vi "Split_Head_Tail.vi"(5 "Number of Cores":i32, 7 "Size":cluster{"X":i32, "Y":i32}, 9 "Major Angle":dbl, 10 "Centroid":cluster{"X":dbl, "Y":dbl}, 11 "Image Pixels (single)":sgl[][](array[numeric])) -> (1 "P2":sgl[][](array[numeric]), 2 "P1":sgl[][](array[numeric]), 3 "Split Line Points":cluster{"X":i32, "Y":i32}[](array[cluster]))   [LabVIEW 2014]
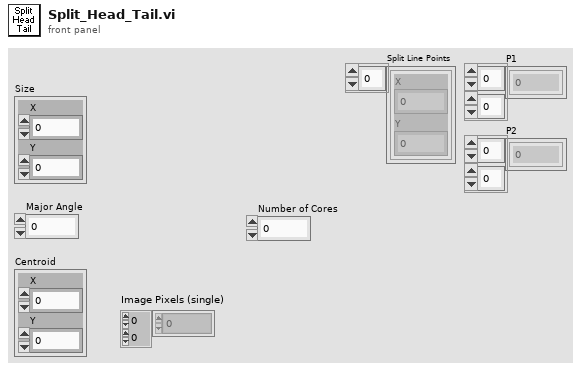
[diagram p1: front panel]
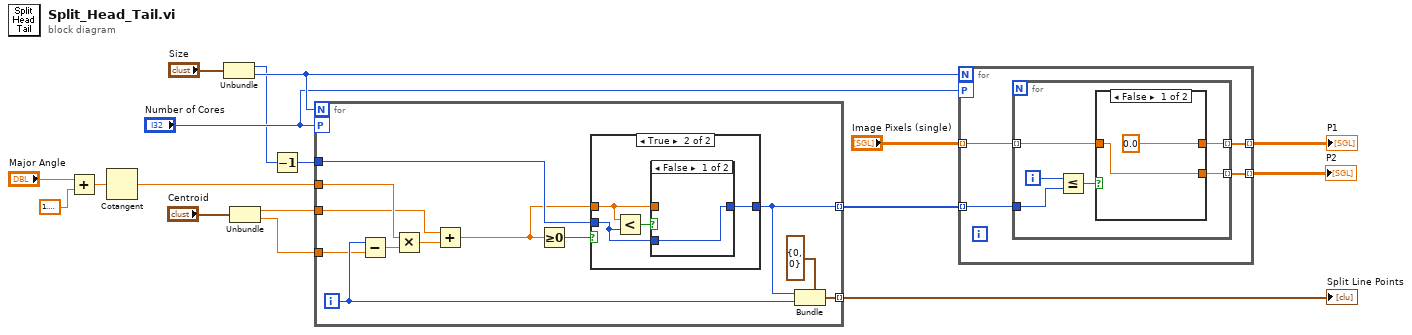
[diagram p0: block diagram]
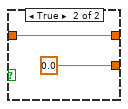
[diagram p2: hidden frame]
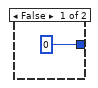
[diagram p3: hidden frame]
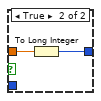
[diagram p4: hidden frame]
diagram:
  n1 = Add(x="Major Angle", y=1.5707963267948966) -> (x+y=w4:dbl)
  n2 = Cotangent(1:w4) -> (0:w3:dbl)
  n3 = Unbundle("Size") -> ("X"=w2:i32, "Y"=w10:i32)
  n4 = Unbundle("Centroid") -> ("X"=w12:dbl, "Y"=w11:dbl)
  n5 = Decrement(x=w2) -> (x-1=w1:i32)
  n6 = for {
    N: w10 -> [_]
    tunnel: w3 -> [w21]
    tunnel: w12 -> [w19]
    tunnel: w11 -> [w23]
    workers-P: "Number of Cores" -> [_]
    tunnel: w1 -> [w27]
    tunnel: [w26] -> w17 mode=indexing
    tunnel: [w25] -> w9 mode=indexing
    i -> [w24]
    n7 = Subtract(x=w24, y=w23) -> (x-y=w22:dbl)
    n8 = Multiply(x=w21, y=w22) -> (x*y=w20:dbl)
    n9 = Add(x=w19, y=w20) -> (x+y=w18:dbl)
    n10 = Greater Or Equal To 0?(x=w18) -> (x >= 0?=w28:bool)
    n11 = case shown="True" w28 {
      tunnel: w18 -> [_ w33]
      tunnel: w27 -> [_ w31]
      tunnel: [0 w32] -> w25
      frame False {
      }
      frame True {
        n12 = Less?(x=w33, y=w31) -> (x < y?=w34:bool)
        n13 = case shown="False" w34 {
          tunnel: w33 -> [_ w37]
          tunnel: [w35 w36] -> w32
          tunnel: w31 -> [w35 _]
          frame False {
          }
          frame True {
            n14 = To Long Integer(number=w37) -> (32bit integer=w36:i32)
          }
        }
      }
    }
    n15 = Bundle(cluster=cluster{"X":i32, "Y":i32} {"X"=0, "Y"=0} ("Start Point"), "X"=w25, "Y"=w24) -> (w26:cluster{"X":i32, "Y":i32})
  }
  "Split Line Points" <- w17
  n16 = for {
    N: w10 -> [_]
    workers-P: "Number of Cores" -> [_]
    tunnel: "Image Pixels (single)" -> [w41] mode=indexing
    tunnel: w9 -> [w40] mode=indexing
    tunnel: [w39] -> w16 mode=indexing
    tunnel: [w38] -> w15 mode=indexing
    n17 = for {
      tunnel: w41 -> [w44] mode=indexing
      tunnel: w40 -> [w46]
      tunnel: [w43] -> w39 mode=indexing
      tunnel: [w42] -> w38 mode=indexing
      i -> [w47]
      n18 = Less Or Equal?(x=w47, y=w46) -> (x <= y?=w45:bool)
      n19 = case shown="False" w45 {
        tunnel: w44 -> [w49 w51]
        tunnel: [sgl 0.0 w51] -> w43
        tunnel: [w49 sgl 0.0] -> w42
        frame False {
        }
        frame True {
        }
      }
    }
  }
  "P1" <- w16
  "P2" <- w15
